vi "GetParam.vi"(8 "error in (no error)":errorcluster caption="entrée d'erreur (pas d'erreur)", 11 "QuantileTransformer.lvclass":refnum<class "QuantileTransformer.lvclass">) -> (0 "error out":errorcluster caption="sortie d'erreur", 2 "QuantileTransformer":T1={"n_quantiles"=1000, "output_distribution"="uniform", "ignore_implicit_zeros"=FALSE, "subsample"=100000.0, "random_state"=-1, "copy"=TRUE} {"random_state" min=-1}, 3 "QuantileTransformer.lvclass":refnum<class "QuantileTransformer.lvclass">)   [LabVIEW 2020, in "QuantileTransformer.lvclass"]
doc: "Get Parameters"
uses:
  QuantileTransformer.lvclass
  QuantileTransformer.lvclass/QuantileTransformer.ctl
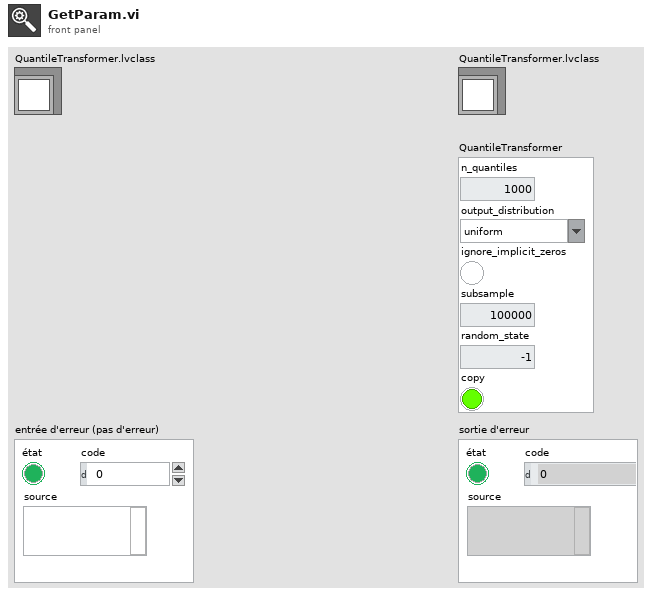
[diagram p1: front panel]
types:
  T1 = cluster{"n_quantiles":i32, "output_distribution":string, "ignore_implicit_zeros":bool, "subsample":dbl, "random_state":i32, "copy":bool}
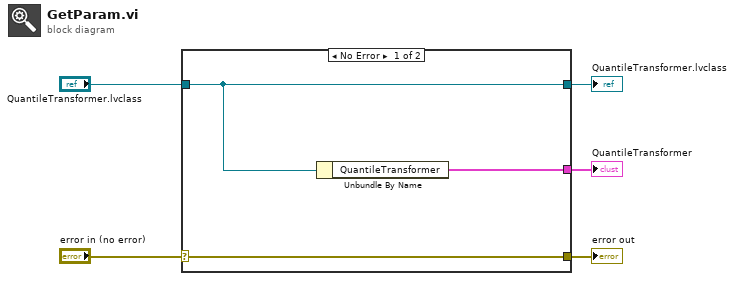
[diagram p0: block diagram]
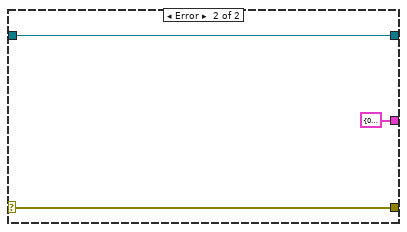
[diagram p2: hidden frame]
diagram:
  n1 = case shown="No Error" "error in (no error)" {
    selector: "error in (no error)" -> [w8 w10]
    tunnel: [w8 w10] -> w4
    tunnel: [w7 w11] -> w2
    tunnel: "QuantileTransformer.lvclass" -> [w7 w11]
    tunnel: [w6 T1 {"n_quantiles"=0, "output_distribution"="", "ignore_implicit_zeros"=FALSE, "subsample"=0.0, "random_state"=0, "copy"=FALSE} ("QuantileTransformer")] -> w1
    frame No Error {
      n2 = Unbundle By Name(w7) -> ("QuantileTransformer"=w6:T1)
    }
    frame Error {
    }
  }
  "error out" <- w4
  "QuantileTransformer.lvclass" <- w2
  "QuantileTransformer" <- w1
